vi "SV Test for Measurement Settled (1 Ch) (Waveform) (DBL).vi"(8 "error in (no error)":errorcluster, 10 "settling configuration":T1={"target value"=inf, "tolerance"=1.0, "units"=1, "time constant [s]"=0.0, "mask duration [s]"=0.0} {"target value" format="%_4g"; "mask duration [s]" min=-1.0 step=0.1 format="%_4g"; "time constant [s]" format="%_4g"; "units" items=["Input units", "% of target"]; "tolerance" format="%_4g"}, 11 "waveform data in":waveform(dbl)) -> (0 "error out":errorcluster, 1 "output values":waveform(dbl)[](graph), 2 "point results":bool[](array[boolean]), 3 "settled?":bool)   [LabVIEW 2017]
doc: "Use this VI to test a settled double-precision output of an input array or waveform. Use the <B>settling configuration</B> input to configure the settling mask parameters. <B>output values</B> returns the thresholds and failures from the settling mask. Use the waveform instance of this VI to test waveform input."
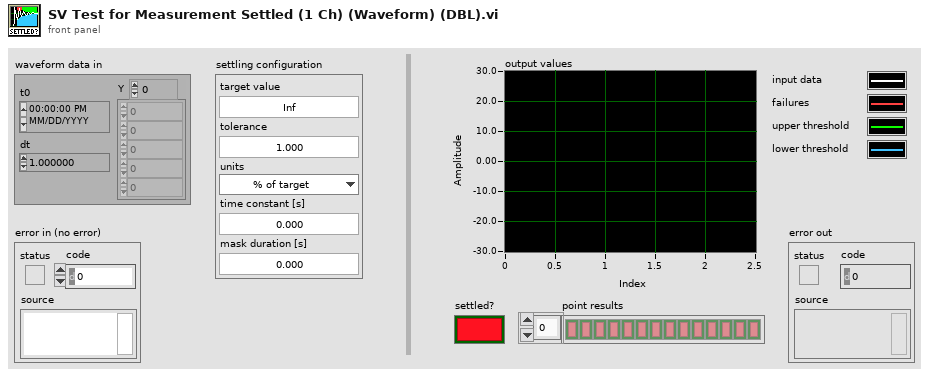
[diagram p1: front panel]
types:
  T1 = cluster{"target value":dbl, "tolerance":dbl, "units":u16, "time constant [s]":dbl, "mask duration [s]":dbl}
  T2 = cluster{"target value":dbl, "tolerance":dbl, "units":u16, "normalized time constant\n[samples]":dbl, "mask length [samples]":i32}
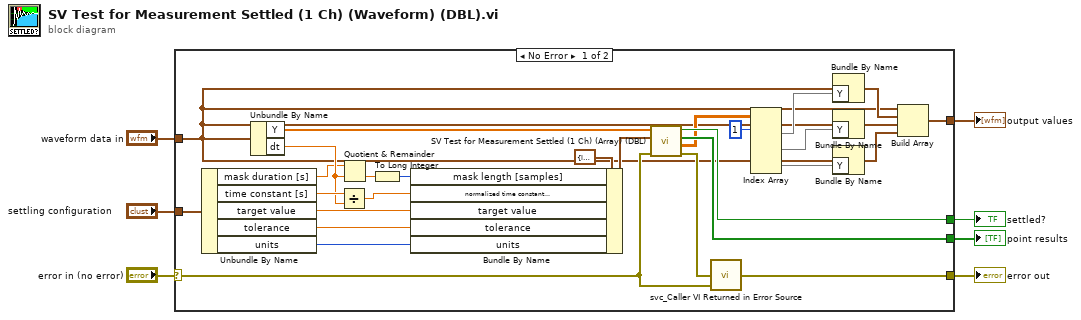
[diagram p0: block diagram]
diagram:
  n1 = case shown="No Error" "error in (no error)" {
    selector: "error in (no error)" -> [w26 w36]
    tunnel: [w33 _] -> w7
    tunnel: [w32 _] -> w6
    tunnel: "waveform data in" -> [w9 _]
    tunnel: [w8 _] -> w4
    tunnel: [w35 w36] -> w2
    tunnel: "settling configuration" -> [w31 _]
    frame No Error {
      n2 = Unbundle By Name(w31) -> ("mask duration [s]"=w20:dbl, "time constant [s]"=w23:dbl, "target value"=w29:dbl, "tolerance"=w25:dbl, "units"=w24:u16)
      n3 = Unbundle By Name(w9) -> ("Y"=w34:dbl[], "dt"=w21:dbl)
      n4 = Divide(x=w23, y=w21) -> (x/y=w22:dbl)
      n5 = Quotient & Remainder(x=w20, y=w21) -> (floor(x/y)=w19:dbl)  [unwired: 1 out]
      n6 = To Long Integer(number=w19) -> (32bit integer=w18:i32)
      n7 = Bundle By Name(cluster=T2 {"target value"=inf, "tolerance"=1.0, "units"=1, "normalized time constant\n[samples]"=0.0, "mask length [samples]"=0} ("settling configuration"), "mask length [samples]"=w18, "normalized time constant\n[samples]"=w22, "target value"=w29, "tolerance"=w25, "units"=w24) -> (w28:T2)
      n8 = call <vilib>:"SV Test for Measurement Settled (1 Ch) (Array) (DBL).vi"("error in (no error)"=w26, "settling configuration"=w28, "data in"=w34) -> ("error out"=w27:errorcluster, "output values"=w17:dbl[][], "point results"=w32:bool[], "settled?"=w33:bool)  [unwired: 5 in]
      n9 = call <vilib>:"svc_Caller VI Returned in Error Source.vi"("warning input to caller"=w26, "error in (no error)"=w27) -> ("error out"=w35:errorcluster)  [unwired: 3 in]
      n10 = Index Array(array=w17, index (row) #1=1 ("index (row)")) -> (element #1=w16:dbl[], element #2=w14:dbl[], element #3=w13:dbl[])  [unwired: 5 in]
      n11 = Bundle By Name(cluster=w9, "Y"=w16) -> (w12:waveform(dbl))
      n12 = Bundle By Name(cluster=w9, "Y"=w14) -> (w11:waveform(dbl))
      n13 = Bundle By Name(cluster=w9, "Y"=w13) -> (w10:waveform(dbl))
      n14 = Build Array(w9, w12, w11, w10) -> (w8:waveform(dbl)[])
    }
    frame Error {
    }
  }
  "settled?" <- w7
  "point results" <- w6
  "output values" <- w4
  "error out" <- w2
